vi "TX JESD.vi"(0 "txjesd.control":T1, 5 "trigger value":bool) -> ()   [LabVIEW 2019]
uses:
  <vilib>/rvi/eio/common/nirviEmuTemplateMethod_errors.vi
  <vilib>/eio/EIONode/EIONode.xnode
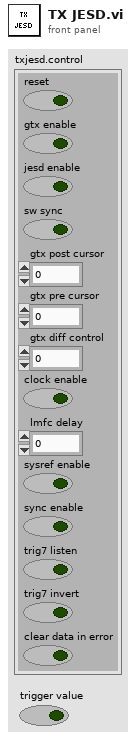
[diagram p1: front panel]
types:
  T1 = cluster{"reset":bool, "gtx enable":bool, "jesd enable":bool, "sw sync":bool, "gtx post cursor":fxp<+,5,5>, "gtx pre cursor":fxp<+,5,5>, "gtx diff control":fxp<+,4,4>, "clock enable":bool, "lmfc delay":fxp<+,5,5>, "sysref enable":bool, "sync enable":bool, "trig7 listen":bool, "trig7 invert":bool, "clear data in error":bool}
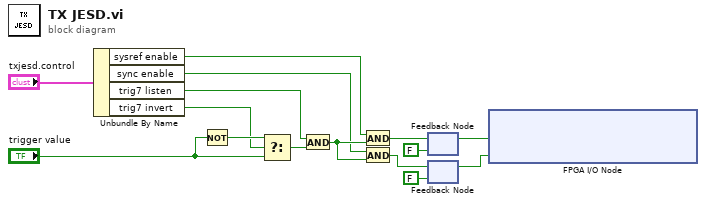
[diagram p0: block diagram]
diagram:
  n1 = Unbundle By Name("txjesd.control") -> ("sysref enable"=w6:bool, "sync enable"=w5:bool, "trig7 listen"=w4:bool, "trig7 invert"=w3:bool)
  n2 = Not(x="trigger value") -> (.not. x?=w11:bool)
  n3 = Select(t=w11, s=w3, f="trigger value") -> (s? t:f=w8:bool)
  n4 = And(x=w4, y=w8) -> (x .and. y?=w7:bool)
  n5 = And(x=w6, y=w7) -> (x .and. y?=w15:bool)
  n6 = And(x=w5, y=w7) -> (x .and. y?=w12:bool)
  n7 = feedback #1(FALSE) -> (w14:bool)
  n8 = feedback-in #1(w15) -> ()
  n9 = feedback #2(FALSE) -> (w13:bool)
  n10 = feedback-in #2(w12) -> ()
  n11 = xnode "FPGA I/O Node"("7902R IO Socket\\aSysRef"=w14, "7902R IO Socket\\aSyncFromPin"=w13) -> ()  [unwired: 2 in, 2 out]
